vi "Analiza algorytmu przetwarzania wolnego.vi"() -> ()   [LabVIEW 2014]
uses:
  Kontrolki/GUI/RejWol_typ.ctl
  <vilib>/measure/NI_MABase.lvlib
panel:
  in  "frequency":dbl=50.0 format="%#_13g"
  out "Œrednia":dbl
  out "Wyprostowana":dbl
  out "size(s)":i32
  out "dt":dbl
  out "ABS Mean (DC)":dbl
  out "ABS Cycle Average":dbl
  out "RMS":dbl
  out "Mean (DC)":dbl
  out "Cycle RMS":dbl
  out "Cycle Average":dbl
  in  "amplitude":dbl=1.0 format="%0.2p"
  in  "offset":dbl format="%0.2p"
  in  "signal type":T1(ring)
  out "Sygna³ testowy":waveform(dbl)[](graph)
  out "Skuteczna":dbl
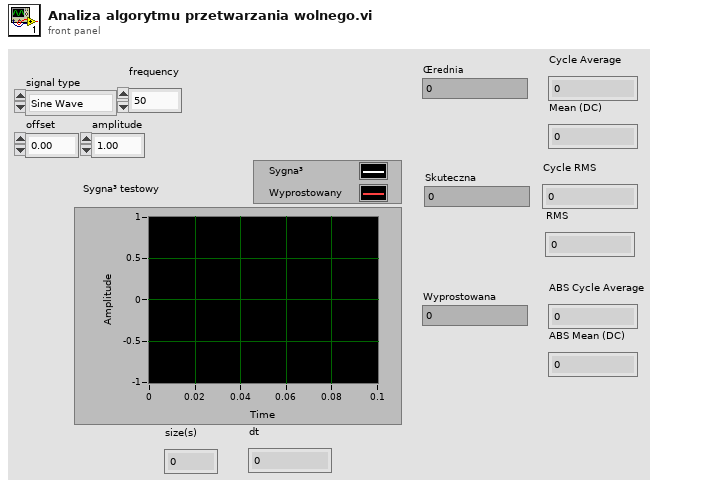
[diagram p1: front panel]
types:
  T1 = enum16{"Sine Wave", "Triangle Wave", "Square Wave", "Sawtooth Wave"}
  T2 = typedef "RejWol_typ.ctl" = enum16{"Wprost (œrednia)", "Modu³ (œr. wypr)", "Kwadrat (skuteczna)", "Iloczyn", "Faza"}
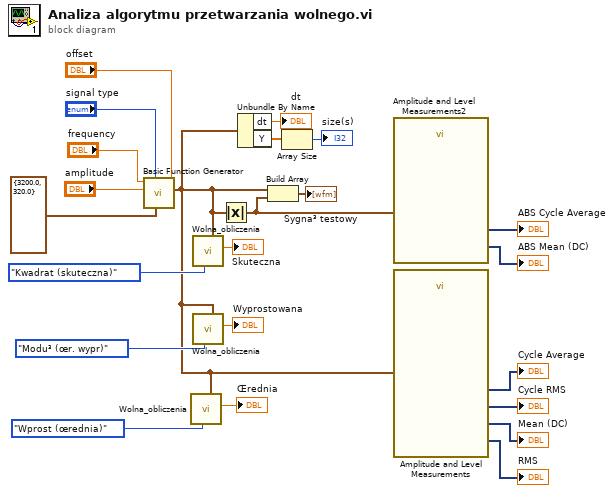
[diagram p0: block diagram]
diagram:
  n1 = call <vilib>:"Basic Function Generator.vi"("offset"="offset", "sampling info"=cluster{"Fs":dbl, "#s":dbl} {"Fs"=3200.0, "#s"=320.0}, "signal type"="signal type", "amplitude"="amplitude", "frequency"="frequency") -> ("signal out"=w1:waveform(dbl))  [unwired: 4 in, 2 out]
  n2 = call "Wolna_obliczenia.vi"("Wektor1 in"=w1, "Typ rejestracji"=RejWol_typ."Wprost (œrednia)") -> ("Value out"=→"Œrednia":dbl)  [unwired: 7 in, 2 out]
  n3 = call "Wolna_obliczenia.vi"("Wektor1 in"=w1, "Typ rejestracji"=RejWol_typ."Kwadrat (skuteczna)") -> ("Value out"=→"Skuteczna":dbl)  [unwired: 7 in, 2 out]
  n4 = call "Wolna_obliczenia.vi"("Wektor1 in"=w1, "Typ rejestracji"=RejWol_typ."Modu³ (œr. wypr)") -> ("Value out"=→"Wyprostowana":dbl)  [unwired: 7 in, 2 out]
  n5 = Absolute Value(x=w1) -> (abs(x)=w16:waveform(dbl))
  n6 = Unbundle By Name(w1) -> ("dt"=→"dt":dbl, "Y"=w8:dbl[])
  n7 = Build Array(w1, w16) -> (→"Sygna³ testowy":waveform(dbl)[])
  n8 = Array Size(array=w8) -> (size(s)=→"size(s)":i32)
  n9 = call "Amplitude and Level Measurements2"("Signals"=w16) -> ("Cycle Average"=→"ABS Cycle Average":dynamicdata, "Mean (DC)"=→"ABS Mean (DC)":dynamicdata)  [unwired: 12 in, 1 out]
  n10 = call "Amplitude and Level Measurements"("Signals"=w1) -> ("Cycle Average"=→"Cycle Average":dynamicdata, "Cycle RMS"=→"Cycle RMS":dynamicdata, "Mean (DC)"=→"Mean (DC)":dynamicdata, "RMS"=→"RMS":dynamicdata)  [unwired: 10 in, 1 out]
